vi "PID Controller.vi"(8 "error in (no error)":errorcluster, 11 "Node Ptr":T1 format="%.0x") -> (0 "error out":errorcluster)   [LabVIEW 2019, in "Control Addon System Explorer.lvlib"]
uses:
  Control Addon System Explorer.lvlib
  <vilib>/NI VeriStand/Custom Device API/Custom Device Item Ref.ctl
  NationalInstruments.VeriStand.SystemStorageUI
  Types/Action.ctl
  Addon Shared/Constants.vi
  <vilib>/NI VeriStand/Custom Device API/NI VeriStand - Get Item Property.vi
  <vilib>/NI VeriStand/Custom Device API/Get Item Property (Double).vi
  <vilib>/NI VeriStand/Custom Device API/Get Item Property (Boolean).vi
  <vilib>/NI VeriStand/Custom Device API/NI VeriStand - Set Item Property.vi
  <vilib>/NI VeriStand/Custom Device API/Set Item Property (Double).vi
  <vilib>/NI VeriStand/Custom Device API/Set Item Property (Boolean).vi
  <vilib>/NI VeriStand/UI Controls/Single Node Browser/Register Callbacks.vi
  <vilib>/NI VeriStand/Custom Device Tools/Custom Device Utility Library/NI VeriStand - Search for Item.vi
  <vilib>/NI VeriStand/Custom Device Tools/Custom Device Utility Library/NI VeriStand - Search for Item by GUID.vi
  <vilib>/NI VeriStand/Custom Device API/NI VeriStand - Add Custom Device Channel.vi
  <vilib>/NI VeriStand/Custom Device API/NI VeriStand - Remove Custom Device Item.vi
  <vilib>/NI VeriStand/Custom Device API/Custom Device API.lvlib
  Addon Shared/Control Addon Shared.lvlib
panel:
  in  "Output Rate Limiter":dbl=10.0 caption="Output Rate Limiter (EU/sec)"
  in  "Description":string
  in  "Header 4":cluster{"Section Name":string}={"Section Name"="Setpoint Signal Settings"}
  in  "Header 3":cluster{"Section Name":string}={"Section Name"="Output Signal Settings"}
  in  "Header 2":cluster{"Section Name":string}={"Section Name"="Feedback Signal Settings"}
  in  "Setpoint Min":dbl caption="Setpoint Min (EU)"
  in  "Setpoint Max":dbl caption="Setpoint Max (EU)"
  in  "Output Min":dbl caption="Output Min (EU)"
  in  "Output Max":dbl caption="Output Max (EU)"
  in  "Setpoint":refnum<k24>(container)
  in  "Use External Setpoint":bool
  in  "Output":refnum<k24>(container)
  in  "Feedback":refnum<k24>(container)
  in  "SHDocVw.IWebBrowser":refnum<k7>(container)
  in  "Header":cluster{"Section Name":string}={"Section Name"="Custom Device Item Settings"}
  in  "Name":string
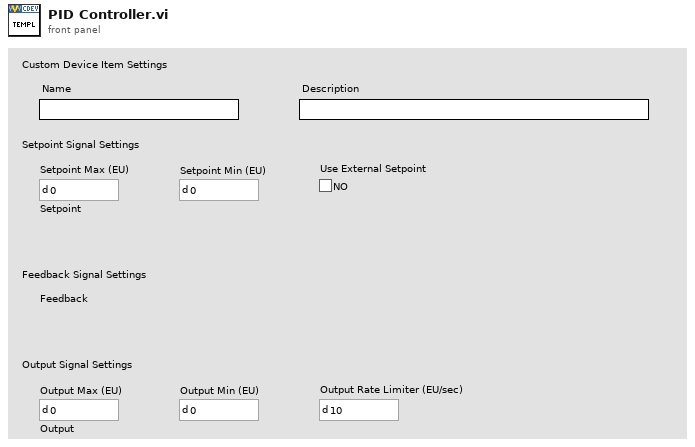
[diagram p1: front panel]
types:
  T1 = typedef "Custom Device API.lvlib/Custom Device Item Ref.ctl" = u64
  T2 = typedef "Control Addon System Explorer.lvlib/Action.ctl" = enum16{"Get", "Set"}
  T3 = typedef "Control Addon Shared.lvlib/Controller Settings.ctl" = cluster{"Output Max":dbl, "Output Min":dbl, "Setpoint Max":dbl, "Setpoint Min":dbl, "Use External Setpoint":bool, "Output Rate Limiter":dbl}
  T4 = typedef "Control Addon System Explorer.lvlib/PID Controller Channel Browser Refs.ctl" = cluster{"Output":refnum<user-event>, "Setpoint":refnum<user-event>, "Feedback":refnum<user-event>}
  T5 = typedef "Custom Device API.lvlib/Custom Device Item Info.ctl" = cluster{"Name":string, "Is Channel":bool, "GUID":string, "Is Waveform":bool}
  T6 = typedef "Custom Device API.lvlib/Custom Device Commands.ctl" = enum16{"Default", "Item renamed", "Shutdown", "Dynamic button pressed"}
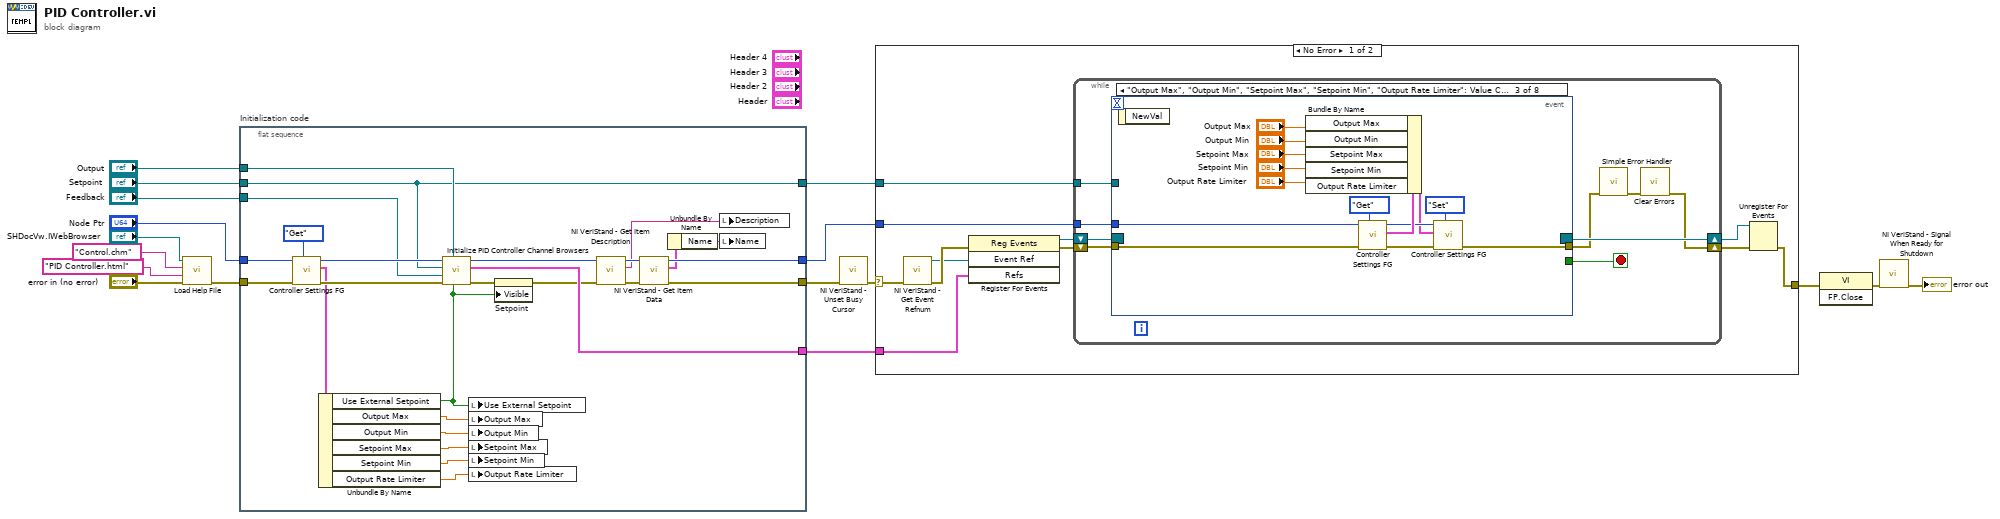
[diagram p0: block diagram]
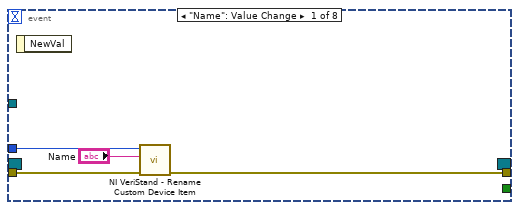
[diagram p2: hidden frame]
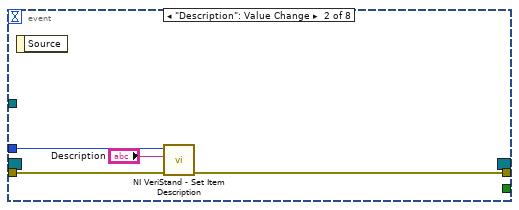
[diagram p3: hidden frame]
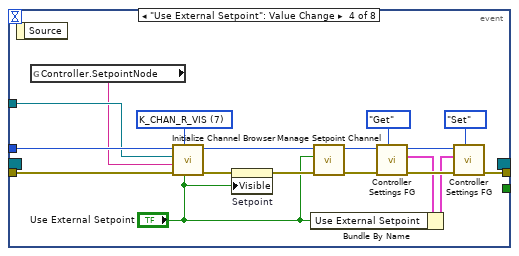
[diagram p4: hidden frame]
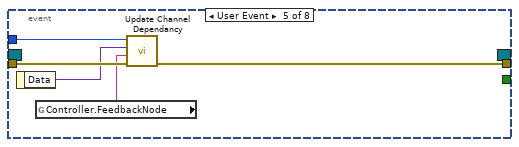
[diagram p5: hidden frame]
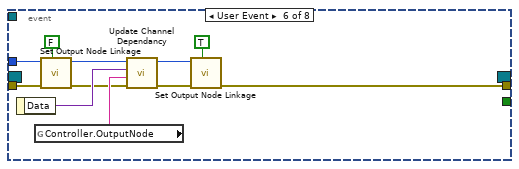
[diagram p6: hidden frame]
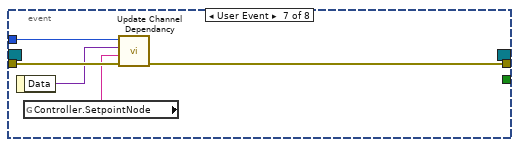
[diagram p7: hidden frame]
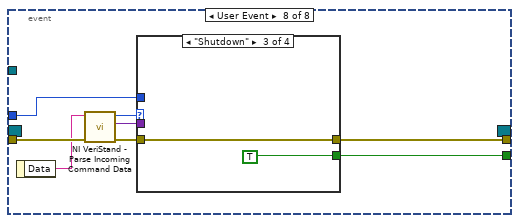
[diagram p8: hidden frame]
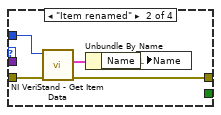
[diagram p10: hidden frame]
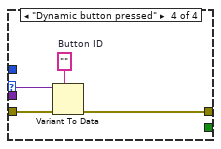
[diagram p11: hidden frame]
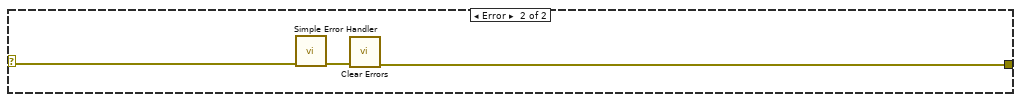
[diagram p12: hidden frame]
diagram:
  n1 = call "Load Help File.vi"("error in (no error)"="error in (no error)", "HTML File"="PID Controller.html", "Main CHM File"="Control.chm", "SHDocVw.IWebBrowser2"="SHDocVw.IWebBrowser") -> ("error out"=w9:errorcluster)  [unwired: 7 in]
  n2 = flat-sequence "Initialization code" {
    tunnel: w9 -> [w35]
    tunnel: "Node Ptr" -> [w34]
    tunnel: [w37] -> w13
    tunnel: [w43] -> w11
    tunnel: [w25] -> w5
    tunnel: [w20] -> w4
    tunnel: "Output" -> [w21]
    tunnel: "Setpoint" -> [w20]
    tunnel: "Feedback" -> [w19]
    frame #0 {
      n3 = call "Controller Settings FG.vi"("Action"=Action."Get", "error in (no error)"=w35, "Node Ptr"=w34) -> ("error out"=w32:errorcluster, "Controller Settings"=w30:T3, "Item Ref out"=w33:T1)  [unwired: 6 in]
      n4 = Unbundle By Name(w30) -> ("Use External Setpoint"=w22:bool, "Output Max"=w29:dbl, "Output Min"=w28:dbl, "Setpoint Max"=w27:dbl, "Setpoint Min"=w26:dbl, "Output Rate Limiter"=w18:dbl)
      n5 = call "Initialize PID Controller Channel Browsers.vi"("Use External Setpoint"=w22, "Output"=w21, "error in (no error)"=w32, "Feedback"=w19, "Setpoint in"=w20, "Item Ref in"=w33) -> ("error out"=w24:errorcluster, "Refs"=w25:T4, "Item Ref out"=w36:T1)  [unwired: 3 in]
      n6 = local write "Use External Setpoint"(w22) -> ()
      n7 = local write "Output Max"(w29) -> ()
      n8 = local write "Output Min"(w28) -> ()
      n9 = local write "Setpoint Max"(w27) -> ()
      n10 = local write "Setpoint Min"(w26) -> ()
      n11 = local write "Output Rate Limiter"(w18) -> ()
      n12 = property on="Setpoint" class="AXCont"(error in=w24, "Visible"=w22) -> (error out=w23:errorcluster)  [unwired: 1 in, 1 out]
      n13 = call <vilib>:"NI VeriStand - Get Item Description.vi"("error in (no error)"=w23, "Item Ref in"=w36) -> ("error out"=w40:errorcluster, "Description"=w41:string, "Item Ref out"=w42:T1)  [unwired: 7 out]
      n14 = call <vilib>:"NI VeriStand - Get Item Data.vi"("error in (no error)"=w40, "Item Ref in"=w42) -> ("error out"=w37:errorcluster, "Item Info"=w39:T5, "Item Ref out"=w43:T1)  [unwired: 7 out]
      n15 = Unbundle By Name(w39) -> ("Name"=w38:string)
      n16 = local write "Description"(w41) -> ()
      n17 = local write "Name"(w38) -> ()
    }
  }
  n18 = call <vilib>:"NI VeriStand - Unset Busy Cursor.vi"("error in (no error)"=w13) -> ("error out"=w12:errorcluster)  [unwired: 10 out]
  n19 = case shown="No Error" w12 {
    selector: w12 -> [w46 w147]
    tunnel: [w51 w145] -> w17
    tunnel: w11 -> [w47 _]
    tunnel: w5 -> [w44 _]
    tunnel: w4 -> [w45 _]
    frame No Error {
      n20 = call <vilib>:"NI VeriStand - Get Event Refnum.vi"("error in (no error)"=w46) -> ("error out"=w54:errorcluster, "Event Ref"=w50:refnum<user-event>)  [unwired: 9 out]
      n21 = register-events(error in=w54, w50, w44) -> (reference out=w48:refnum<event-registration>, error out=w49:errorcluster)  [unwired: 1 in]
      n22 = while {
        tunnel: w47 -> [w59]
        shift-right: [w56] -> w52
        shift-left: w49 -> [w62]
        shift-right: [w63] -> w53
        shift-left: w48 -> [w61]
        tunnel: w45 -> [w55]
        stop <- w60 stop-if-true
        n23 = event shown="[2] \"Output Max\", \"Output Min\", \"Setpoint Max\", \"Setpoint Min\", \"Output Rate Limiter\": Value Change" {
          selector: w61 -> [_ _ _ _ _ _ _ _]
          dyn-events: [_ _ _ _ _ _ _ _] -> w63
          timeout: _ -> [_ _ _ _ _ _ _ _]
          tunnel: w62 -> [w67 w70 w84 w96 w108 w113 w124 w132]
          tunnel: [_ _ _ _ _ _ _ w128] -> w60
          tunnel: [w66 w69 w77 w99 w107 w109 w123 w127] -> w58
          tunnel: w59 -> [w65 w71 w83 w95 w106 w112 w122 w126]
          tunnel: w55 -> [_ _ _ w93 _ _ _ _]
          event "Name": Value Change {
            n24 = event-data() -> ()  [unwired: 2 out]
            n25 = call <vilib>:"NI VeriStand - Rename Custom Device Item.vi"("error in (no error)"=w67, "New Name"="Name", "Item Ref in"=w65) -> ("error out"=w66:errorcluster)  [unwired: 1 in, 7 out]
          }
          event "Description": Value Change {
            n26 = event-data() -> ()  [unwired: 2 out]
            n27 = call <vilib>:"NI VeriStand - Set Item Description.vi"("error in (no error)"=w70, "Description"="Description", "Item Ref in"=w71) -> ("error out"=w69:errorcluster)  [unwired: 8 out]
          }
          event "Output Max", "Output Min", "Setpoint Max", "Setpoint Min", "Output Rate Limiter": Value Change {
            n28 = event-data() -> ()  [unwired: 2 out]
            n29 = call "Controller Settings FG.vi"("Action"=Action."Get", "error in (no error)"=w84, "Node Ptr"=w83) -> ("error out"=w79:errorcluster, "Controller Settings"=w82:T3, "Item Ref out"=w80:T1)  [unwired: 6 in]
            n30 = Bundle By Name(cluster=w82, "Output Max"="Output Max", "Output Min"="Output Min", "Setpoint Max"="Setpoint Max", "Setpoint Min"="Setpoint Min", "Output Rate Limiter"="Output Rate Limiter") -> (w78:T3)
            n31 = call "Controller Settings FG.vi"("Action"=Action."Set", "error in (no error)"=w79, "Controller Settings"=w78, "Node Ptr"=w80) -> ("error out"=w77:errorcluster)  [unwired: 5 in, 2 out]
          }
          event "Use External Setpoint": Value Change {
            w94 = u8 7 items=["K_CHAN_R", "K_CHAN_W", "K_CHAN_RW", "K_CHAN_VOLT", "K_CHAN_FAULT", "K_ALL", "K_CUSTOM", "K_CHAN_R_VIS", "K_CHAN_W_VIS", "K_CHAN_RW_VIS", "K_CHAN_VOLT_VIS", "K_CHAN_FAULT_VIS"] ("DisplayFilter")
            n32 = event-data() -> ()  [unwired: 2 out]
            n33 = global read "Constants.vi" "Controller.SetpointNode"() -> (w86:string)
            n34 = call "Initialize Channel Browser.vi"("Use Channel?"="Use External Setpoint", "DisplayFilter"=w94, "error in (no error)"=w96, "NodeName"=w86, "Browser Ref"=w93, "Item Ref in"=w95) -> ("error out"=w89:errorcluster, "Item Ref out"=w92:T1)  [unwired: 3 in, 1 out]
            n35 = property on="Setpoint" class="AXCont"(error in=w89, "Visible"="Use External Setpoint") -> (error out=w88:errorcluster)  [unwired: 1 in, 1 out]
            n36 = call "Manage Setpoint Channel.vi"("error in (no error)"=w88, "Use External Setpoint"="Use External Setpoint", "Node Ptr"=w92) -> ("error out"=w90:errorcluster, "Node Ptr out"=w91:T1)  [unwired: 7 in]
            n37 = call "Controller Settings FG.vi"("Action"=Action."Get", "error in (no error)"=w90, "Node Ptr"=w91) -> ("error out"=w100:errorcluster, "Controller Settings"=w98:T3, "Item Ref out"=w101:T1)  [unwired: 6 in]
            n38 = Bundle By Name(cluster=w98, "Use External Setpoint"="Use External Setpoint") -> (w97:T3)
            n39 = call "Controller Settings FG.vi"("Action"=Action."Set", "error in (no error)"=w100, "Controller Settings"=w97, "Node Ptr"=w101) -> ("error out"=w99:errorcluster)  [unwired: 5 in, 2 out]
          }
          event User Event {
            n40 = event-data() -> ("Data"=w105:variant)  [unwired: 1 out]
            n41 = global read "Constants.vi" "Controller.FeedbackNode"() -> (w104:string)
            n42 = call "Update Channel Dependancy.vi"("error in (no error)"=w108, "NodeName"=w104, "Data"=w105, "Item Ref in"=w106) -> ("error out"=w107:errorcluster)  [unwired: 6 in, 1 out]
          }
          event User Event {
            n43 = event-data() -> ("Data"=w119:variant)  [unwired: 1 out]
            n44 = global read "Constants.vi" "Controller.OutputNode"() -> (w118:string)
            n45 = call "Set Output Node Linkage.vi"("Add?"=FALSE, "error in"=w113, "Section Ref in"=w112) -> ("error out"=w111:errorcluster, "Item Ref out"=w110:T1)  [unwired: 7 in]
            n46 = call "Update Channel Dependancy.vi"("error in (no error)"=w111, "NodeName"=w118, "Data"=w119, "Item Ref in"=w110) -> ("error out"=w117:errorcluster, "Item Ref out"=w116:T1)  [unwired: 6 in]
            n47 = call "Set Output Node Linkage.vi"("Add?"=TRUE, "error in"=w117, "Section Ref in"=w116) -> ("error out"=w109:errorcluster)  [unwired: 7 in, 1 out]
          }
          event User Event {
            n48 = event-data() -> ("Data"=w121:variant)  [unwired: 1 out]
            n49 = global read "Constants.vi" "Controller.SetpointNode"() -> (w120:string)
            n50 = call "Update Channel Dependancy.vi"("error in (no error)"=w124, "NodeName"=w120, "Data"=w121, "Item Ref in"=w122) -> ("error out"=w123:errorcluster)  [unwired: 6 in, 1 out]
          }
          event User Event {
            n51 = event-data() -> ("Data"=w131:string)  [unwired: 1 out]
            n52 = call <vilib>:"NI VeriStand - Parse Incoming Command Data.vi"("error in (no error)"=w132, "Incoming data"=w131) -> ("error out"=w130:errorcluster, "Outgoing data"=w125:variant, "Action"=w129:T6)  [unwired: 7 out]
            n53 = case shown="\"Shutdown\"" w129 {
              tunnel: w130 -> [w133 w138 w139 w144]
              tunnel: [_ _ TRUE _] -> w128
              tunnel: [w133 w135 w139 w141] -> w127
              tunnel: w126 -> [_ w137 _ _]
              tunnel: w125 -> [_ _ _ w143]
              frame "Default", Default {
              }
              frame "Item renamed" {
                n54 = call <vilib>:"NI VeriStand - Get Item Data.vi"("error in (no error)"=w138, "Item Ref in"=w137) -> ("error out"=w135:errorcluster, "Item Info"=w136:T5)  [unwired: 8 out]
                n55 = Unbundle By Name(w136) -> ("Name"=w134:string)
                n56 = local write "Name"(w134) -> ()
              }
              frame "Shutdown" {
              }
              frame "Dynamic button pressed" {
                w142 = ""  # Button ID
                n57 = Variant To Data(error in=w144, type=w142, Variant=w143) -> (error out=w141:errorcluster)  [unwired: 1 out]
              }
            }
          }
        }
        n58 = call <vilib>:"Simple Error Handler.vi"("error in (no error)"=w58) -> ("error out"=w57:errorcluster)  [unwired: 1 in, 7 out]
        n59 = call <vilib>:"Clear Errors.vi"("error in (no error)"=w57) -> ("error out"=w56:errorcluster)  [unwired: 1 in, 5 out]
      }
      n60 = Unregister For Events(event registration refnum=w53, error in=w52) -> (error out=w51:errorcluster)
    }
    frame Error {
      n61 = call <vilib>:"Simple Error Handler.vi"("error in (no error)"=w147) -> ("error out"=w146:errorcluster)  [unwired: 1 in, 7 out]
      n62 = call <vilib>:"Clear Errors.vi"("error in (no error)"=w146) -> ("error out"=w145:errorcluster)  [unwired: 1 in, 5 out]
    }
  }
  n63 = invoke class="VI" method="FP.Close"(error in=w17) -> (error out=w16:errorcluster)  [unwired: 2 in, 2 out]
  n64 = call <vilib>:"NI VeriStand - Signal When Ready for Shutdown.vi"("error in (no error)"=w16) -> ("error out"=→"error out":errorcluster)  [unwired: 10 out]
